vi "CRUDE_OIL.vi"() -> ()   [LabVIEW 2017]
panel:
  out "CRUDE LIVE PRICE UPDATE":dbl
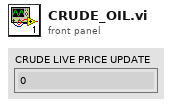
[diagram p1: front panel]
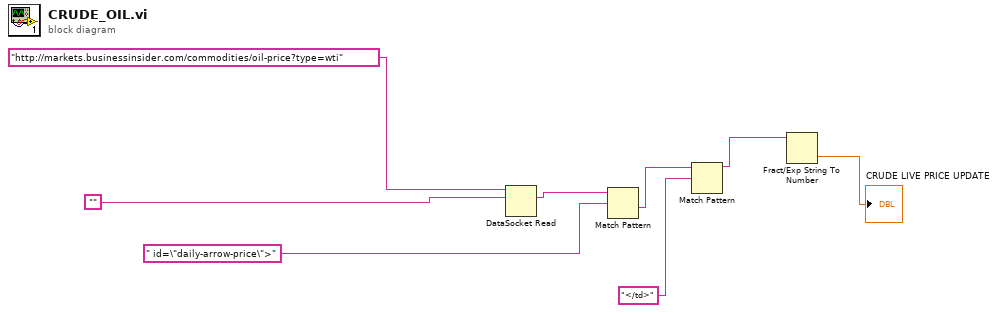
[diagram p0: block diagram]
diagram:
  n1 = DataSocket Read(10:"", 11:"http://markets.businessinsider.com/commodities/oil-price?type=wti") -> (2:w6:string)  [unwired: 3 in, 6 out]
  n2 = Match Pattern(string=w6, regular expression=" id=\"daily-arrow-price\">") -> (after substring=w4:string)  [unwired: 1 in, 3 out]
  n3 = Match Pattern(string=w4, regular expression="</td>") -> (before substring=w2:string)  [unwired: 1 in, 3 out]
  n4 = Fract/Exp String To Number(string=w2) -> (number=→"CRUDE LIVE PRICE UPDATE":dbl)  [unwired: 3 in, 1 out]
